vi "oa_Check Vector Data for Waveform Reference (N Channels).vi"(0 "resampled signal":cluster{"r0":dbl, "dr":dbl, "Y":dbl[]}[](array[cluster]) {"r0" format="%.2p"; "dr" format="%.2p"; "Y" format="%.2f"}, 1 "reset? (True)":bool=TRUE, 5 "slow roll vectors":cdb[][](array[numeric]) format="%.2f", 7 "orders to compensate":dbl[](array[numeric])=[1.0] format="%.2f", 11 "error out in":errorcluster) -> (2 "empty signal?":bool, 3 "parameter changed":bool, 4 "resampled signal dup":cluster{"r0":dbl, "dr":dbl, "Y":dbl[]}[](array[cluster]) {"r0" format="%.2p"; "dr" format="%.2p"; "Y" format="%.2f"}, 6 "slow roll vectors dup":cdb[][](array[numeric]) format="%.2f", 8 "orders to compensate dup":dbl[](array[numeric])=[1.0] format="%.2f", 15 "error out":errorcluster)   [LabVIEW 2017, in "SoundVib_RefDataProcess.lvlib"]
uses:
  <vilib>/addons/Sound and Vibration/Order Analysis/Referece Data Processing/SoundVib_RefDataProcess.lvlib
  <vilib>/addons/Sound and Vibration/Order Analysis/Resample Order Tracking/SubVIs/OAT Verify Resampled Signal (Multi Channels).vi
  <vilib>/addons/Sound and Vibration/Order Analysis/Resample Order Tracking/SoundVib_Resampling.lvlib
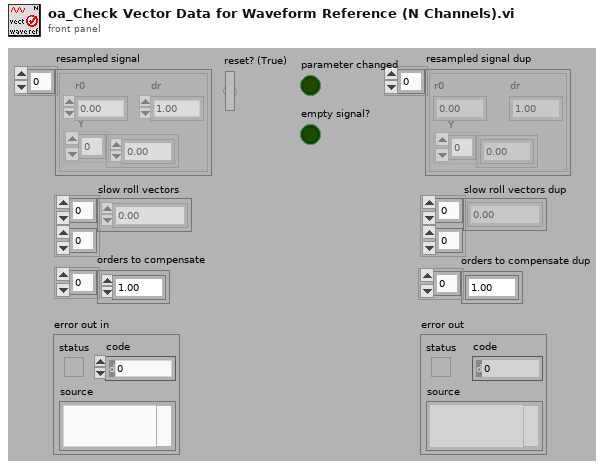
[diagram p1: front panel]
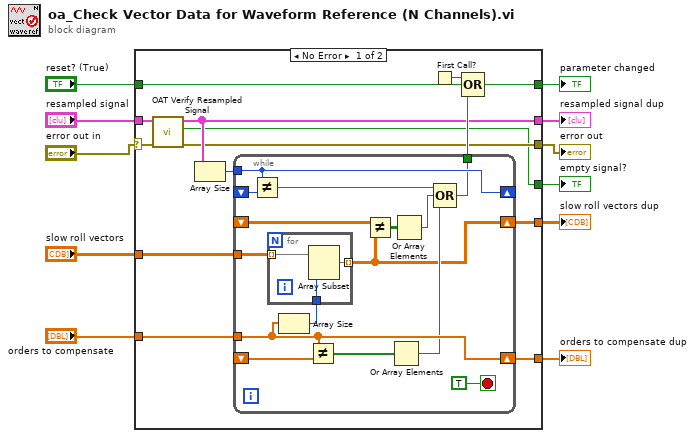
[diagram p0: block diagram]
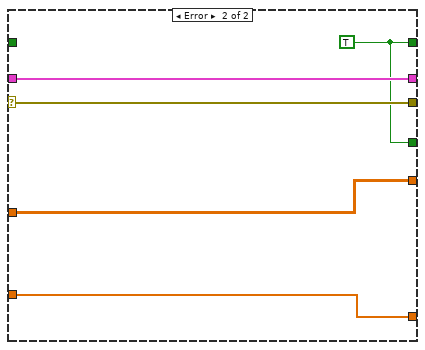
[diagram p2: hidden frame]
diagram:
  n1 = case shown="No Error" "error out in" {
    selector: "error out in" -> [w14 w48]
    tunnel: [w13 w48] -> w10
    tunnel: "resampled signal" -> [w16 w45]
    tunnel: [w15 w45] -> w8
    tunnel: "slow roll vectors" -> [w25 w46]
    tunnel: "orders to compensate" -> [w24 w47]
    tunnel: "reset? (True)" -> [w21 _]
    tunnel: [w20 w44] -> w4
    tunnel: [w19 w46] -> w3
    tunnel: [w18 w47] -> w2
    tunnel: [w12 w44] -> w1
    frame No Error {
      n2 = call-poly <vilib>:"OAT Verify Resampled Signal.vi"("error in (no error)"=w14, "resampled signal"=w16) -> ("error out"=w13:errorcluster, "empty signal"=w12:bool, "resampled signal out"=w15:cluster{"r0":dbl, "dr":dbl, "Y":dbl[]}[])  [unwired: 7 in]
      n3 = Array Size(array=w15) -> (size(s)=w23:i32)
      n4 = while {
        tunnel: w25 -> [w35]
        tunnel: w24 -> [w39]
        shift-right: [w39] -> w18
        shift-left: _ -> [w38]
        shift-right: [w27] -> w19
        shift-left: _ -> [w36]
        tunnel: w23 -> [w33]
        shift-right: [w33] -> _
        shift-left: _ -> [w32]
        tunnel: [w28] -> w22
        stop <- TRUE stop-if-true
        n5 = Not Equal?(x=w33, y=w32) -> (x != y?=w31:bool)
        n6 = Array Size(array=w39) -> (size(s)=w26:i32)
        n7 = for {
          tunnel: w35 -> [w43] mode=indexing
          tunnel: [w42] -> w27 mode=indexing
          tunnel: w26 -> [w41]
          n8 = Array Subset(array=w43, length=w41) -> (w42:cdb[])  [unwired: 1 in]
        }
        n9 = Not Equal?(x=w39, y=w38) -> (x != y?=w37:bool[])
        n10 = Not Equal?(x=w36, y=w27) -> (x != y?=w34:bool[][])
        n11 = Or Array Elements(Boolean array=w37) -> (logical OR=w29:bool)
        n12 = Or Array Elements(Boolean array=w34) -> (logical OR=w30:bool)
        n13 = Compound Arithmetic op=OR(w31, w30, w29) -> (w28:bool)
      }
      n14 = First Call?() -> (First Call?: T/F=w17:bool)
      n15 = Compound Arithmetic op=OR(w17, w21, w22) -> (w20:bool)
    }
    frame Error {
      w44 = TRUE
    }
  }
  "resampled signal dup" <- w8
  "error out" <- w10
  "slow roll vectors dup" <- w3
  "orders to compensate dup" <- w2
  "parameter changed" <- w4
  "empty signal?" <- w1
